vi "cw_1_4.vi"() -> ()   [LabVIEW 2022 SP3]
panel:
  out "Out":dbl
  in  "In":dbl
  in  "Enum":enum16{"F -> C", "C -> F"}(ring)
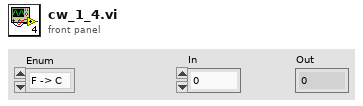
[diagram p1: front panel]
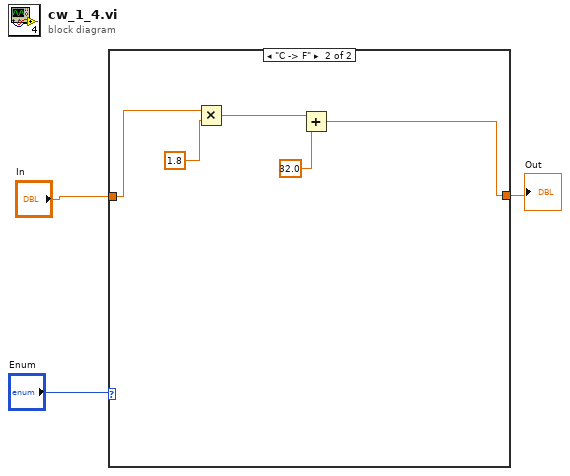
[diagram p0: block diagram]
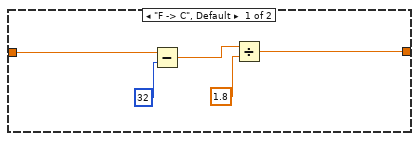
[diagram p2: hidden frame]
diagram:
  n1 = case shown="\"C -> F\"" "Enum" {
    tunnel: "In" -> [w5 w10]
    tunnel: [w4 w9] -> w1
    frame "F -> C", Default {
      n2 = Subtract(x=w5, y=32) -> (x-y=w6:dbl)
      n3 = Divide(x=w6, y=1.8) -> (x/y=w4:dbl)
    }
    frame "C -> F" {
      n4 = Multiply(x=w10, y=1.8) -> (x*y=w12:dbl)
      n5 = Add(x=w12, y=32.0) -> (x+y=w9:dbl)
    }
  }
  "Out" <- w1
